vi "Write File.vi"(4 "Data Column Headings":string[](array[string]), 6 "Write Last Run? (F)":bool, 7 "Current Scan #":u32, 8 "error in":errorcluster, 9 "Data Store":T1, 10 "#scans":u32, 11 "File IO in":refnum<class "File IO.lvclass">) -> (0 "errorOUT":errorcluster, 3 "File IO out":refnum<class "File IO.lvclass">)   [LabVIEW 2012, in "File IO.lvclass"]
uses:
  File IO.lvclass
  Instruments/Utility Classes/Readable/Data Store.ctl
  Instruments/Utility Classes/Readable/Data Point.ctl
  Instruments/Utility Classes/Readable/Time.ctl
  Instruments/Utility Classes/Readable/X.ctl
  File IO.lvclass/File IO.ctl
  Instruments/Utility Classes/Readable/Readable.lvclass
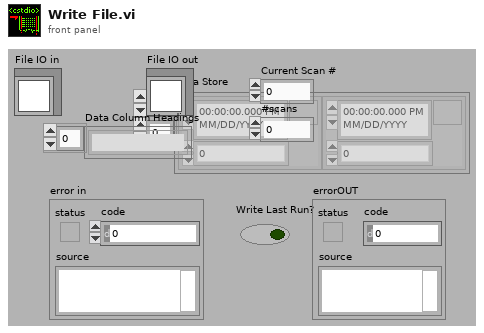
[diagram p1: front panel]
types:
  T1 = typedef "Readable.lvclass/Data Store.ctl" = T2[][]
  T2 = typedef "Readable.lvclass/Data Point.ctl" = cluster{"t":T3, "x":T4}
  T3 = typedef "Readable.lvclass/Time.ctl" = timestamp
  T4 = typedef "Readable.lvclass/X.ctl" = dbl
  T5 = enum16{"open", "replace", "create", "open or create", "replace or create", "replace or create with confirmation"}
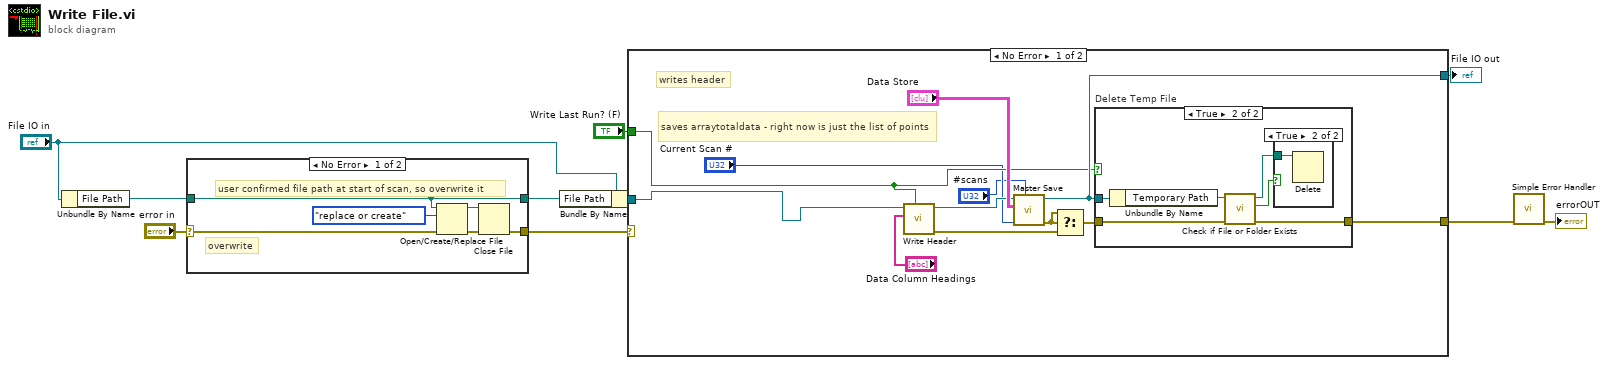
[diagram p0: block diagram]
diagram:
  n1 = Unbundle By Name("File IO in") -> ("File Path"=w2:path)
  n2 = case shown="No Error" "error in" {
    selector: "error in" -> [w13 w17]
    tunnel: w2 -> [w11 w18]
    tunnel: [w11 w18] -> w3
    tunnel: [w12 w17] -> w9
    frame No Error {
      # "overwrite"
      # "user confirmed file path at start of scan, so overwrite it"
      n3 = Open/Create/Replace File(file path (use dialog)=w11, error in=w13, operation (0:open)=T5."replace or create") -> (refnum out=w16:refnum<file>, error out=w15:errorcluster)  [unwired: 4 out]
      n4 = Close File(refnum=w16, error in=w15) -> (error out=w12:errorcluster)  [unwired: 1 out]
    }
    frame Error {
      # "User cancelled?"
    }
  }
  n5 = Bundle By Name(cluster="File IO in", "File Path"=w3) -> (w4:refnum<class "File IO.lvclass">)
  n6 = case shown="No Error" w9 {
    selector: w9 -> [_ w40]
    tunnel: [w26 w39] -> w8
    tunnel: "Write Last Run? (F)" -> [w23 _]
    tunnel: [w24 w40] -> w6
    tunnel: w4 -> [w19 w39]
    frame No Error {
      # "saves arraytotaldata - right now is just the list of points"
      # "writes header"
      n7 = call "Write Header.vi"("Record this scan as \"last run\"?"=w23, "Data Column Headings"="Data Column Headings", "File IO in"=w19) -> ("errorOUT"=w27:errorcluster, "File IO out"=w29:refnum<class "File IO.lvclass">)  [unwired: 2 in, 5 out]
      n8 = call "Master Save.vi"("#scans"="#scans", "Current Scan #"="Current Scan #", "Data Store"="Data Store", "File IO in"=w29) -> ("error out"=w28:errorcluster, "File IO out"=w26:refnum<class "File IO.lvclass">)  [unwired: 6 out]
      n9 = Select(t=w28, s=w28, f=w27) -> (s? t:f=w25:errorcluster)
      n10 = case "Delete Temp File" shown="True" w23 {
        tunnel: w26 -> [_ w33]
        tunnel: w25 -> [w31 w35]
        tunnel: [w31 w34] -> w24
        frame False {
        }
        frame True {
          n11 = Unbundle By Name(w33) -> ("Temporary Path"=w32:path)
          n12 = call <vilib>:"Check if File or Folder Exists.vi"("error in (no error)"=w35, "path"=w32) -> ("error out"=w34:errorcluster, "file or folder exists?"=w36:bool, "dup path"=w37:path)  [unwired: 7 out]
          n13 = case shown="True" w36 {
            tunnel: w37 -> [_ w38]
            frame False {
            }
            frame True {
              n14 = Delete(path (use dialog)=w38) -> ()  [unwired: 1 in, 6 out]
            }
          }
        }
      }
    }
    frame Error {
    }
  }
  "File IO out" <- w8
  n15 = call <vilib>:"Simple Error Handler.vi"("error in (no error)"=w6) -> ("error out"=→"errorOUT":errorcluster)  [unwired: 1 in, 7 out]
